vi "PI_AreaScan_Prepare_1.vi"(0 "System":i32 min=0 max=3 step=1, 1 "Laser":string="1", 2 "Axis":string="xy", 3 "da":dbl min=-100.0 max=100.0, 4 "db":dbl min=-100.0 max=100.0, 5 "error in (no error)":errorcluster caption="Fehler (Eingang, kein Fehler)", 6 "a0":dbl=98.0 min=2.0 max=198.0 step=0.01, 8 "b0":dbl min=0.0 max=200.0 step=0.01, 9 "Resolution":dbl=0.01 min=0.01 max=2.0 step=0.01, 10 "c0":dbl min=0.0 max=200.0 step=0.01, 11 "Pixel time":dbl) -> (14 "Tacq":dbl, 15 "lp":i32, 16 "ap":i32, 17 "Trigger":dbl[](array[numeric]), 19 "error out":errorcluster caption="Fehler (Ausgang)")   [LabVIEW 2013]
panel:
  out "ClockDivider":i32
  out "Amplitude":dbl format="%#_3g"
  out "Accelaration":dbl
  out "ttp":i32
  out "Scan lines":dbl
  out "slow axis":i32
  out "fast axis":i32
  out "Colors":i32
  out "Start position":dbl[](array[numeric])
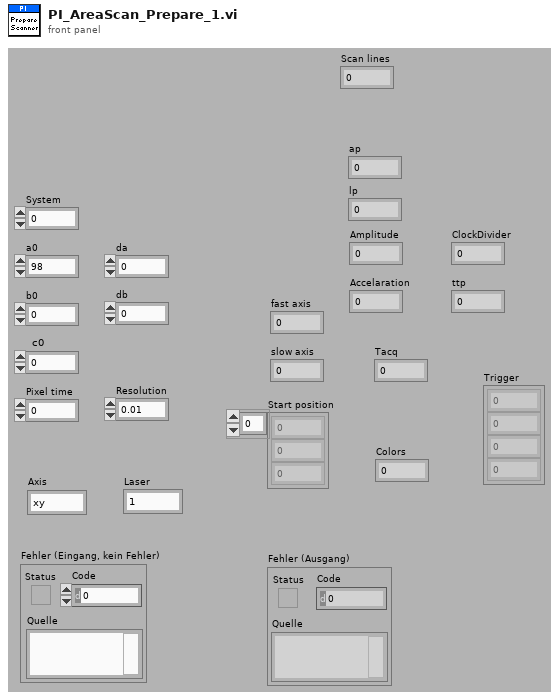
[diagram p1: front panel]
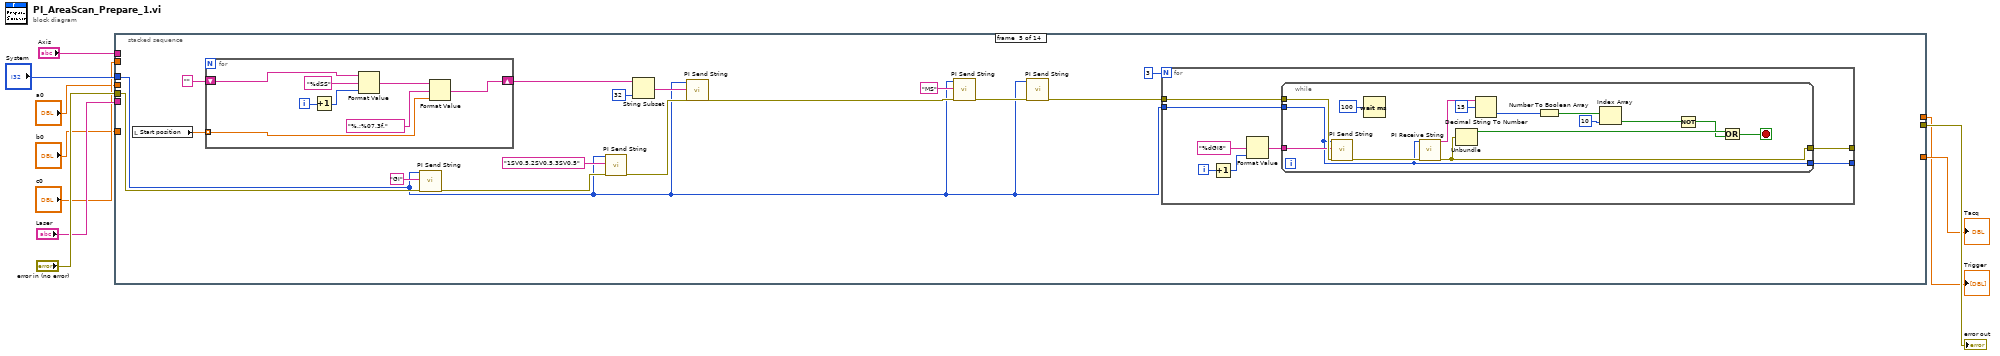
[diagram p0: block diagram]
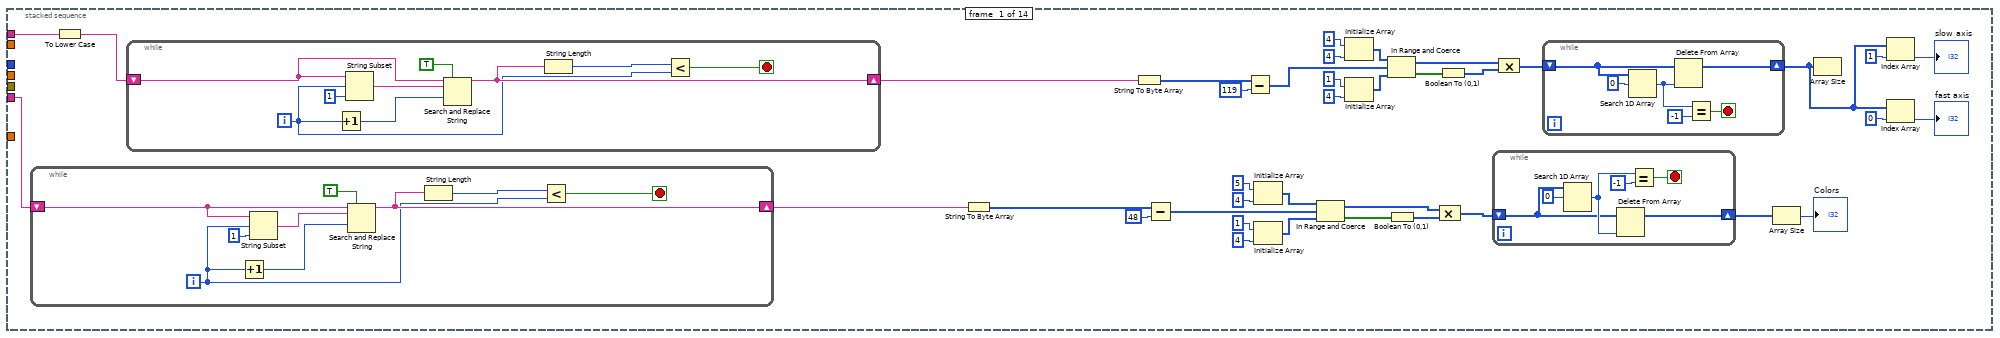
[diagram p2: hidden frame]
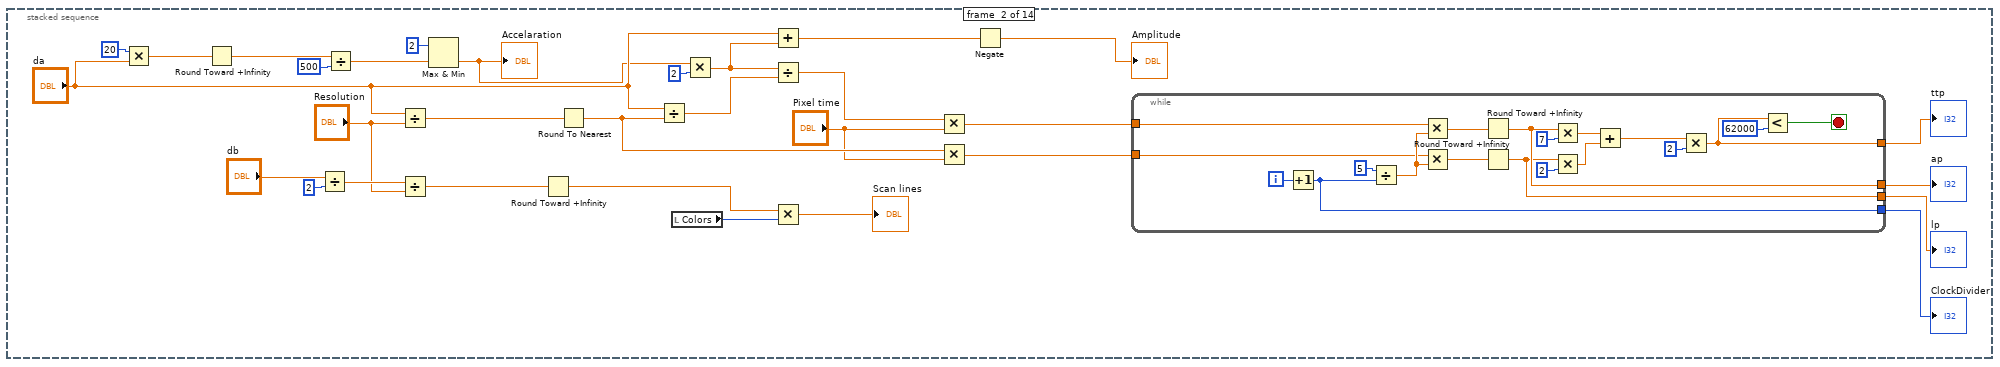
[diagram p3: hidden frame]
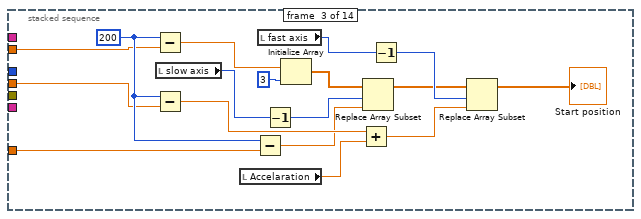
[diagram p4: hidden frame]
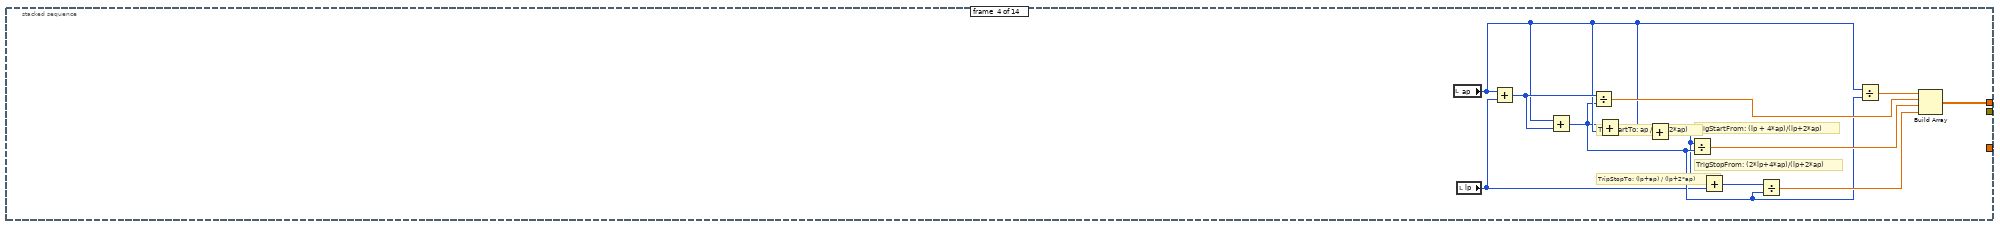
[diagram p5: hidden frame]
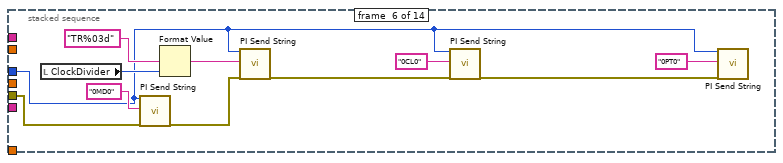
[diagram p6: hidden frame]
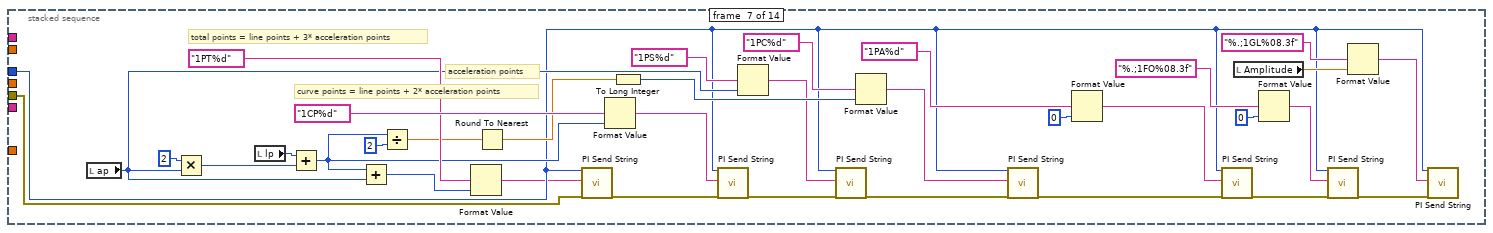
[diagram p7: hidden frame]
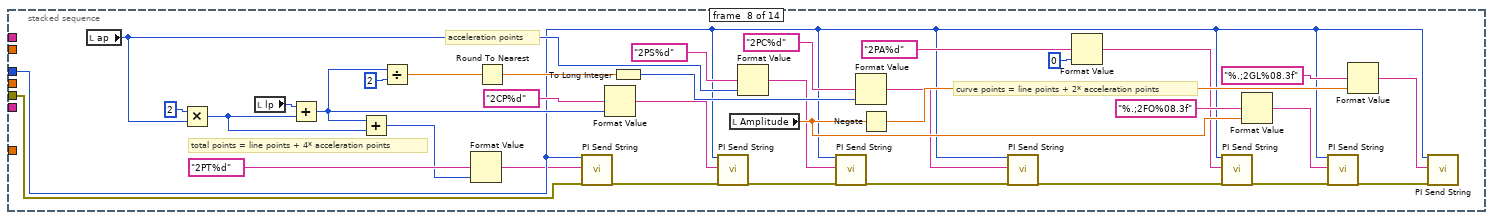
[diagram p8: hidden frame]
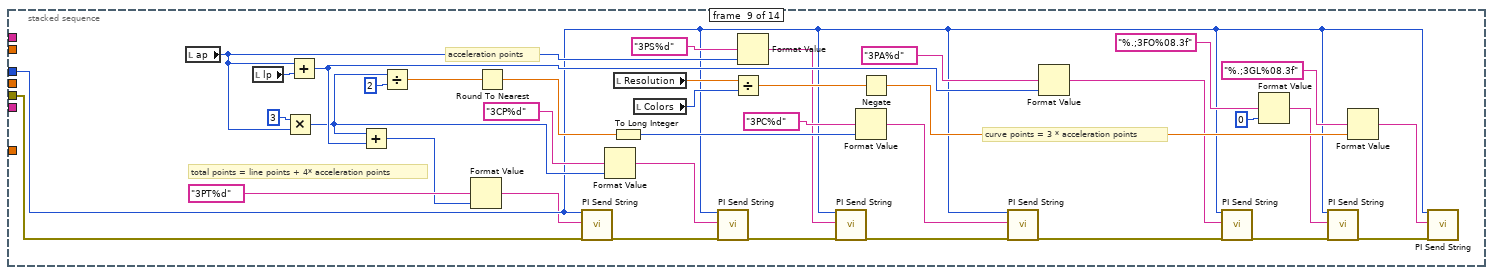
[diagram p9: hidden frame]
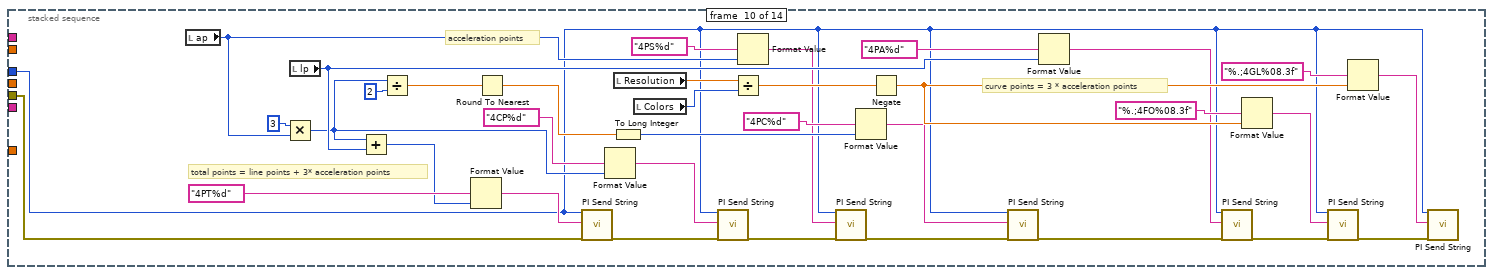
[diagram p10: hidden frame]
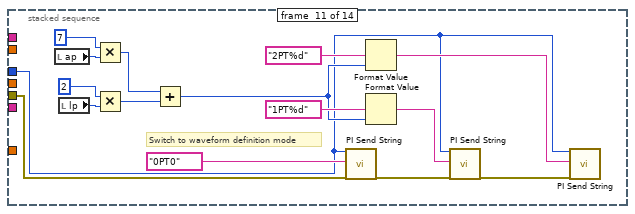
[diagram p11: hidden frame]
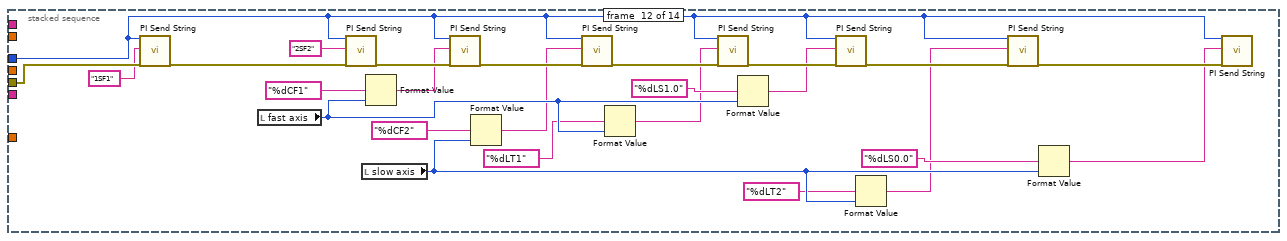
[diagram p12: hidden frame]
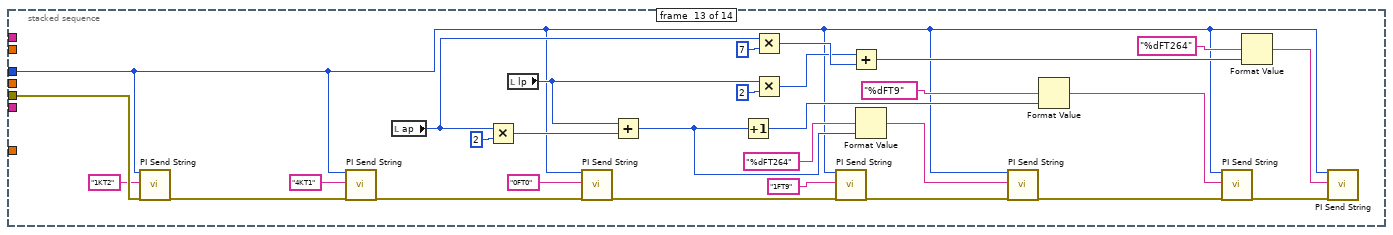
[diagram p13: hidden frame]
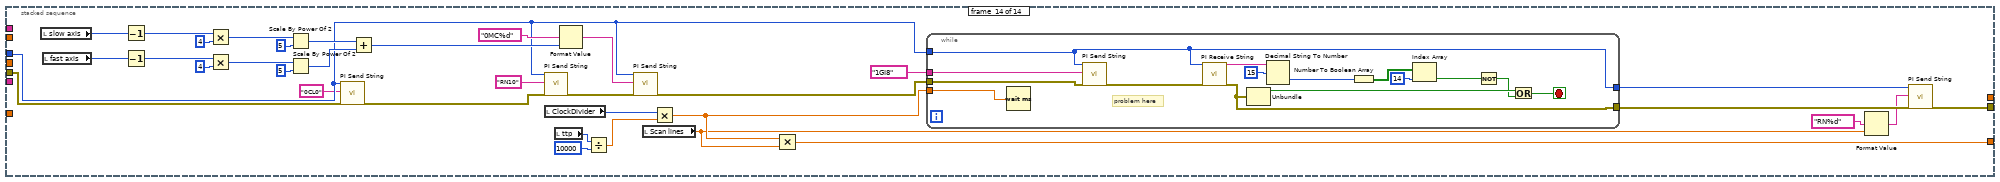
[diagram p14: hidden frame]
diagram:
  n1 = stacked-sequence {
    tunnel: "System" -> [_ _ _ _ w159 w207 w223 w258 w293 w323 w358 w374 w399 w435]
    tunnel: "error in (no error)" -> [_ _ _ _ w167 w212 w224 w265 w300 w331 w362 w390 w407 w439]
    tunnel: [_ _ _ _ _ _ _ _ _ _ _ _ _ w428] -> w8
    tunnel: "Laser" -> [w12 _ _ _ _ _ _ _ _ _ _ _ _ _]
    tunnel: "Axis" -> [w11 _ _ _ _ _ _ _ _ _ _ _ _ _]
    tunnel: "c0" -> [_ _ w131 _ _ _ _ _ _ _ _ _ _ _]
    tunnel: "b0" -> [_ _ w130 _ _ _ _ _ _ _ _ _ _ _]
    tunnel: "a0" -> [_ _ w129 _ _ _ _ _ _ _ _ _ _ _]
    tunnel: [_ _ _ _ _ _ _ _ _ _ _ _ _ w440] -> w2
    tunnel: [_ _ _ w146 _ _ _ _ _ _ _ _ _ _] -> w1
    frame #0 {
      n2 = while {
        shift-right: [w74] -> w39
        shift-left: w12 -> [w78]
        i -> [w70]
        stop <- w73 stop-if-true
        n3 = Increment(x=w70) -> (x+1=w71:i32)
        n4 = String Subset(string=w78, offset (0)=w70, length (rest)=1) -> (substring=w76:string)
        n5 = Search and Replace String(replace all?=TRUE, input string=w78, search string=w76, offset=w71) -> (result string=w74:string)  [unwired: 4 in, 3 out]
        n6 = String Length(string=w74) -> (length=w72:i32)
        n7 = Less?(x=w72, y=w70) -> (x < y?=w73:bool)
      }
      n8 = To Lower Case(string=w11) -> (all lower case string=w19:string)
      n9 = while {
        shift-right: [w59] -> w24
        shift-left: w19 -> [w63]
        i -> [w55]
        stop <- w58 stop-if-true
        n10 = Increment(x=w55) -> (x+1=w56:i32)
        n11 = String Subset(string=w63, offset (0)=w55, length (rest)=1) -> (substring=w61:string)
        n12 = Search and Replace String(replace all?=TRUE, input string=w63, search string=w61, offset=w56) -> (result string=w59:string)  [unwired: 4 in, 3 out]
        n13 = String Length(string=w59) -> (length=w57:i32)
        n14 = Less?(x=w57, y=w55) -> (x < y?=w58:bool)
      }
      n15 = String To Byte Array(string=w39) -> (unsigned byte array=w41:u8[])
      n16 = String To Byte Array(string=w24) -> (unsigned byte array=w26:u8[])
      n17 = Subtract(x=w41, y=48) -> (x-y=w38:i32[])
      n18 = Subtract(x=w26, y=119) -> (x-y=w23:i32[])
      n19 = Initialize Array(5, 4) -> (w46:i32[])
      n20 = Initialize Array(1, 4) -> (w43:i32[])
      n21 = In Range and Coerce(upper limit=w46, x=w38, lower limit=w43) -> (coerced(x)=w35:i32[], In Range?=w42:bool[])
      n22 = Initialize Array(4, 4) -> (w31:i32[])
      n23 = Initialize Array(1, 4) -> (w28:i32[])
      n24 = In Range and Coerce(upper limit=w31, x=w23, lower limit=w28) -> (coerced(x)=w20:i32[], In Range?=w27:bool[])
      n25 = Boolean To (0,1)(Boolean=w42) -> (0, 1=w36:i16[])
      n26 = Boolean To (0,1)(Boolean=w27) -> (0, 1=w21:i16[])
      n27 = Compound Arithmetic op=MULTIPLY(w35, w36) -> (w37:i32[])
      n28 = while {
        shift-right: [w66] -> w34
        shift-left: w37 -> [w64]
        stop <- w67 stop-if-true
        n29 = Search 1D Array(1D array=w64, element=0) -> (index of element=w68:i32)  [unwired: 1 in]
        n30 = Delete From Array(array=w64, index=w68) -> (array with subset deleted=w66:i32[])  [unwired: 1 in, 1 out]
        n31 = Equal?(x=w68, y=-1) -> (x = y?=w67:bool)
      }
      n32 = Compound Arithmetic op=MULTIPLY(w20, w21) -> (w22:i32[])
      n33 = while {
        shift-right: [w51] -> w16
        shift-left: w22 -> [w49]
        stop <- w52 stop-if-true
        n34 = Search 1D Array(1D array=w49, element=0) -> (index of element=w53:i32)  [unwired: 1 in]
        n35 = Delete From Array(array=w49, index=w53) -> (array with subset deleted=w51:i32[])  [unwired: 1 in, 1 out]
        n36 = Equal?(x=w53, y=-1) -> (x = y?=w52:bool)
      }
      n37 = Array Size(array=w34) -> (size(s)=→"Colors":i32)
      n38 = Array Size(array=w16) -> ()  [unwired: 1 out]
      n39 = Index Array(array=w16, index=1) -> (element=→"slow axis":i32)
      n40 = Index Array(array=w16, index=0) -> (element=→"fast axis":i32)
    }
    frame #1 {
      n41 = Multiply(x=20, y="da") -> (x*y=w108:dbl)
      n42 = Round Toward +Infinity(x=w108) -> (ceil(x): smallest int >= x=w107:dbl)
      n43 = Divide(x="db", y=2) -> (x/y=w101:dbl)
      n44 = Divide(x=w107, y=500) -> (x/y=w105:dbl)
      n45 = Divide(x="da", y="Resolution") -> (x/y=w103:dbl)
      n46 = Divide(x=w101, y="Resolution") -> (x/y=w95:dbl)
      n47 = Max & Min(x=2, y=w105) -> (min(x,y)=w86:dbl)  [unwired: 1 out]
      "Accelaration" <- w86
      n48 = Round Toward +Infinity(x=w95) -> (ceil(x): smallest int >= x=w96:dbl)
      n49 = Round To Nearest(number=w103) -> (nearest integer value=w90:dbl)
      n50 = Divide(x="da", y=w90) -> (x/y=w89:dbl)
      n51 = local read "Colors"() -> (w98:i32)
      n52 = Multiply(x=w86, y=2) -> (x*y=w88:dbl)
      n53 = Add(x="da", y=w88) -> (x+y=w80:dbl)
      n54 = Divide(x=w88, y=w89) -> (x/y=w91:dbl)
      n55 = Multiply(x=w96, y=w98) -> (x*y=→"Scan lines":dbl)
      n56 = Multiply(x=w91, y="Pixel time") -> (x*y=w92:dbl)
      n57 = Multiply(x=w90, y="Pixel time") -> (x*y=w94:dbl)
      n58 = Negate(x=w80) -> (-x=→"Amplitude":dbl)
      n59 = while {
        tunnel: w94 -> [w125]
        tunnel: w92 -> [w124]
        tunnel: [w113] -> w84
        tunnel: [w112] -> w81
        tunnel: [w111] -> w83
        tunnel: [w110] -> w82
        i -> [w128]
        stop <- w114 stop-if-true
        n60 = Increment(x=w128) -> (x+1=w112:i32)
        n61 = Divide(x=5, y=w112) -> (x/y=w126:dbl)
        n62 = Multiply(x=w124, y=w126) -> (x*y=w123:dbl)
        n63 = Multiply(x=w125, y=w126) -> (x*y=w122:dbl)
        n64 = Round Toward +Infinity(x=w123) -> (ceil(x): smallest int >= x=w111:dbl)
        n65 = Round Toward +Infinity(x=w122) -> (ceil(x): smallest int >= x=w110:dbl)
        n66 = Multiply(x=w111, y=7) -> (x*y=w119:dbl)
        n67 = Multiply(x=w110, y=2) -> (x*y=w118:dbl)
        n68 = Add(x=w119, y=w118) -> (x+y=w117:dbl)
        n69 = Multiply(x=w117, y=2) -> (x*y=w113:dbl)
        n70 = Less?(x=w113, y=62000) -> (x < y?=w114:bool)
      }
      "ttp" <- w84
      "ap" <- w83
      "lp" <- w82
      "ClockDivider" <- w81
    }
    frame #2 {
      w132 = 200
      n71 = Subtract(x=w132, y=w131) -> (x-y=w134:dbl)
      n72 = Subtract(x=w132, y=w129) -> (x-y=w140:dbl)
      n73 = local read "slow axis"() -> (w145:i32)
      n74 = local read "Accelaration"() -> (w142:dbl)
      n75 = Subtract(x=w132, y=w130) -> (x-y=w136:dbl)
      n76 = local read "fast axis"() -> (w144:i32)
      n77 = Decrement(x=w145) -> (x-1=w138:i32)
      n78 = Initialize Array(w134, 3) -> (w135:dbl[])
      n79 = Add(x=w140, y=w142) -> (x+y=w141:dbl)
      n80 = Replace Array Subset(array=w135, new element=w136, index=w138) -> (w137:dbl[])
      n81 = Decrement(x=w144) -> (x-1=w139:i32)
      n82 = Replace Array Subset(array=w137, new element=w141, index=w139) -> (→"Start position":dbl[])
    }
    frame #3 {
      # "TrigStopFrom: (2*lp+4*ap)/(lp+2*ap)"
      # "TrigStartFrom: (lp + 4*ap)/(lp+2*ap)"
      # "TripStopTo: (lp+ap) / (lp+2*ap)"
      # "TrigStartTo: ap / (lp+2*ap)"
      n83 = local read "ap"() -> (w152:i32)
      n84 = local read "lp"() -> (w148:i32)
      n85 = Add(x=w152, y=w148) -> (x+y=w153:i32)
      n86 = Add(x=w152, y=w153) -> (x+y=w151:i32)
      n87 = Divide(x=w153, y=w151) -> (x/y=w155:dbl)
      n88 = Add(x=w151, y=w152) -> (x+y=w150:i32)
      n89 = Add(x=w150, y=w152) -> (x+y=w147:i32)
      n90 = Divide(x=w147, y=w151) -> (x/y=w156:dbl)
      n91 = Add(x=w147, y=w148) -> (x+y=w149:i32)
      n92 = Divide(x=w149, y=w151) -> (x/y=w157:dbl)
      n93 = Divide(x=w152, y=w151) -> (x/y=w154:dbl)
      n94 = Build Array(w154, w155, w156, w157) -> (w146:dbl[])
    }
    frame #4 {
      n95 = local read "Start position"() -> (w171:dbl[])
      n96 = for {
        shift-right: [w202] -> w172
        shift-left: "" -> [w204]
        tunnel: w171 -> [w197] mode=indexing
        i -> [w199]
        n97 = Increment(x=w199) -> (x+1=w198:i32)
        n98 = Format Value(string ("")=w204, format string="%dSS", value (0)=w198) -> (output string=w203:string)
        n99 = Format Value(string ("")=w203, format string="%.;%07.3f,", value (0)=w197) -> (output string=w202:string)
      }
      n100 = call "PI Send String.vi"("System no."=w159, "String to send"="GI", "error in"=w167) -> ("error out"=w166:errorcluster)  [unwired: 16 in]
      n101 = call "PI Send String.vi"("System no."=w159, "String to send"="1SV0.5,2SV0.5,3SV0.5", "error in"=w166) -> ("error out"=w163:errorcluster)  [unwired: 16 in]
      n102 = String Subset(string=w172, length (rest)=32) -> (substring=w164:string)  [unwired: 1 in]
      n103 = call "PI Send String.vi"("System no."=w159, "String to send"=w164, "error in"=w163) -> ("error out"=w161:errorcluster)  [unwired: 16 in]
      n104 = call "PI Send String.vi"("System no."=w159, "String to send"="MS", "error in"=w161) -> ("error out"=w160:errorcluster)  [unwired: 16 in]
      n105 = call "PI Send String.vi"("System no."=w159, "error in"=w160) -> ("error out"=w158:errorcluster)  [unwired: 17 in]
      n106 = for {
        N: 3 -> [_]
        tunnel: w158 -> [w177]
        tunnel: w159 -> [w176]
        tunnel: [w175] -> _
        tunnel: [w174] -> _
        i -> [w181]
        n107 = Increment(x=w181) -> (x+1=w180:i32)
        n108 = Format Value(format string="%dGI8", value (0)=w180) -> (output string=w178:string)  [unwired: 1 in]
        n109 = while {
          tunnel: w178 -> [w186]
          tunnel: w177 -> [w187]
          tunnel: w176 -> [w184]
          tunnel: [w182] -> w175
          tunnel: [w184] -> w174
          stop <- w190 stop-if-true
          n110 = call "PI Send String.vi"("System no."=w184, "String to send"=w186, "error in"=w187) -> ("error out"=w185:errorcluster)  [unwired: 16 in]
          n111 = Wait (ms)(milliseconds to wait=100) -> ()  [unwired: 1 out]
          n112 = call "PI Receive String.vi"("System no."=w184, "error in"=w185) -> ("String read"=w183:string, "error out"=w182:errorcluster)  [unwired: 15 in, 1 out]
          n113 = Unbundle(w182) -> ("status"=w194:bool)  [unwired: 2 out]
          n114 = Decimal String To Number(string=w183, offset=15) -> (number=w195:i32)  [unwired: 1 in, 1 out]
          n115 = Number To Boolean Array(number=w195) -> (Boolean array=w192:bool[])
          n116 = Index Array(array=w192, index=10) -> (element=w191:bool)
          n117 = Not(x=w191) -> (.not. x?=w188:bool)
          n118 = Or(x=w194, y=w188) -> (x .or. y?=w190:bool)
        }
      }
    }
    frame #5 {
      n119 = local read "ClockDivider"() -> (w215:i32)
      n120 = call "PI Send String.vi"("System no."=w207, "String to send"="0MD0", "error in"=w212) -> ("error out"=w211:errorcluster)  [unwired: 16 in]
      n121 = Format Value(format string="TR%03d", value (0)=w215) -> (output string=w206:string)  [unwired: 1 in]
      n122 = call "PI Send String.vi"("System no."=w207, "String to send"=w206, "error in"=w211) -> ("error out"=w210:errorcluster)  [unwired: 16 in]
      n123 = call "PI Send String.vi"("System no."=w207, "String to send"="0CL0", "error in"=w210) -> ("error out"=w209:errorcluster)  [unwired: 16 in]
      n124 = call "PI Send String.vi"("System no."=w207, "String to send"="0PT0", "error in"=w209) -> ()  [unwired: 16 in, 1 out]
    }
    frame #6 {
      # "acceleration points"
      # "total points = line points + 3* acceleration points"
      # "curve points = line points + 2* acceleration points"
      n125 = local read "ap"() -> (w239:i32)
      n126 = Multiply(x=2, y=w239) -> (x*y=w242:i32)
      n127 = local read "lp"() -> (w241:i32)
      n128 = Add(x=w241, y=w242) -> (x+y=w236:i32)
      n129 = Add(x=w236, y=w239) -> (x+y=w240:i32)
      n130 = Divide(x=w236, y=2) -> (x/y=w235:dbl)
      n131 = Format Value(format string="1PT%d", value (0)=w240) -> (output string=w222:string)  [unwired: 1 in]
      n132 = Round To Nearest(number=w235) -> (nearest integer value=w232:dbl)
      n133 = call "PI Send String.vi"("System no."=w223, "String to send"=w222, "error in"=w224) -> ("error out"=w230:errorcluster)  [unwired: 16 in]
      n134 = Format Value(format string="1CP%d", value (0)=w236) -> (output string=w221:string)  [unwired: 1 in]
      n135 = To Long Integer(number=w232) -> (32bit integer=w233:i32)
      n136 = call "PI Send String.vi"("System no."=w223, "String to send"=w221, "error in"=w230) -> ("error out"=w229:errorcluster)  [unwired: 16 in]
      n137 = Format Value(format string="1PS%d", value (0)=w239) -> (output string=w220:string)  [unwired: 1 in]
      n138 = call "PI Send String.vi"("System no."=w223, "String to send"=w220, "error in"=w229) -> ("error out"=w228:errorcluster)  [unwired: 16 in]
      n139 = Format Value(format string="1PC%d", value (0)=w233) -> (output string=w219:string)  [unwired: 1 in]
      n140 = call "PI Send String.vi"("System no."=w223, "String to send"=w219, "error in"=w228) -> ("error out"=w227:errorcluster)  [unwired: 16 in]
      n141 = Format Value(format string="1PA%d", value (0)=0) -> (output string=w218:string)  [unwired: 1 in]
      n142 = call "PI Send String.vi"("System no."=w223, "String to send"=w218, "error in"=w227) -> ("error out"=w226:errorcluster)  [unwired: 16 in]
      n143 = local read "Amplitude"() -> (w231:dbl)
      n144 = Format Value(format string="%.;1FO%08.3f", value (0)=0) -> (output string=w217:string)  [unwired: 1 in]
      n145 = call "PI Send String.vi"("System no."=w223, "String to send"=w217, "error in"=w226) -> ("error out"=w225:errorcluster)  [unwired: 16 in]
      n146 = Format Value(format string="%.;1GL%08.3f", value (0)=w231) -> (output string=w216:string)  [unwired: 1 in]
      n147 = call "PI Send String.vi"("System no."=w223, "String to send"=w216, "error in"=w225) -> ()  [unwired: 16 in, 1 out]
    }
    frame #7 {
      # "acceleration points"
      # "total points = line points + 4* acceleration points"
      # "curve points = line points + 2* acceleration points"
      n148 = local read "ap"() -> (w276:i32)
      n149 = Multiply(x=2, y=w276) -> (x*y=w275:i32)
      n150 = local read "lp"() -> (w278:i32)
      n151 = Add(x=w278, y=w275) -> (x+y=w269:i32)
      n152 = Add(x=w269, y=w275) -> (x+y=w277:i32)
      n153 = Divide(x=w269, y=2) -> (x/y=w273:dbl)
      n154 = Format Value(format string="2PT%d", value (0)=w277) -> (output string=w257:string)  [unwired: 1 in]
      n155 = Round To Nearest(number=w273) -> (nearest integer value=w270:dbl)
      n156 = call "PI Send String.vi"("System no."=w258, "String to send"=w257, "error in"=w265) -> ("error out"=w264:errorcluster)  [unwired: 16 in]
      n157 = Format Value(format string="2CP%d", value (0)=w269) -> (output string=w256:string)  [unwired: 1 in]
      n158 = To Long Integer(number=w270) -> (32bit integer=w271:i32)
      n159 = call "PI Send String.vi"("System no."=w258, "String to send"=w256, "error in"=w264) -> ("error out"=w263:errorcluster)  [unwired: 16 in]
      n160 = local read "Amplitude"() -> (w267:dbl)
      n161 = Format Value(format string="2PS%d", value (0)=w276) -> (output string=w255:string)  [unwired: 1 in]
      n162 = call "PI Send String.vi"("System no."=w258, "String to send"=w255, "error in"=w263) -> ("error out"=w262:errorcluster)  [unwired: 16 in]
      n163 = Format Value(format string="2PC%d", value (0)=w271) -> (output string=w254:string)  [unwired: 1 in]
      n164 = Negate(x=w267) -> (-x=w266:dbl)
      n165 = call "PI Send String.vi"("System no."=w258, "String to send"=w254, "error in"=w262) -> ("error out"=w261:errorcluster)  [unwired: 16 in]
      n166 = Format Value(format string="2PA%d", value (0)=0) -> (output string=w253:string)  [unwired: 1 in]
      n167 = call "PI Send String.vi"("System no."=w258, "String to send"=w253, "error in"=w261) -> ("error out"=w260:errorcluster)  [unwired: 16 in]
      n168 = Format Value(format string="%.;2FO%08.3f", value (0)=w267) -> (output string=w252:string)  [unwired: 1 in]
      n169 = call "PI Send String.vi"("System no."=w258, "String to send"=w252, "error in"=w260) -> ("error out"=w259:errorcluster)  [unwired: 16 in]
      n170 = Format Value(format string="%.;2GL%08.3f", value (0)=w266) -> (output string=w251:string)  [unwired: 1 in]
      n171 = call "PI Send String.vi"("System no."=w258, "String to send"=w251, "error in"=w259) -> ()  [unwired: 16 in, 1 out]
    }
    frame #8 {
      # "acceleration points"
      # "total points = line points + 4* acceleration points"
      # "curve points = 3 * acceleration points"
      n172 = local read "ap"() -> (w307:i32)
      n173 = local read "lp"() -> (w310:i32)
      n174 = Multiply(x=3, y=w307) -> (x*y=w302:i32)
      n175 = Add(x=w307, y=w310) -> (x+y=w308:i32)
      n176 = Add(x=w302, y=w308) -> (x+y=w316:i32)
      n177 = Divide(x=w302, y=2) -> (x/y=w306:dbl)
      n178 = Format Value(format string="3PT%d", value (0)=w316) -> (output string=w292:string)  [unwired: 1 in]
      n179 = Round To Nearest(number=w306) -> (nearest integer value=w303:dbl)
      n180 = call "PI Send String.vi"("System no."=w293, "String to send"=w292, "error in"=w300) -> ("error out"=w299:errorcluster)  [unwired: 16 in]
      n181 = Format Value(format string="3CP%d", value (0)=w302) -> (output string=w291:string)  [unwired: 1 in]
      n182 = To Long Integer(number=w303) -> (32bit integer=w304:i32)
      n183 = local read "Resolution"() -> (w315:dbl)
      n184 = local read "Colors"() -> (w312:i32)
      n185 = call "PI Send String.vi"("System no."=w293, "String to send"=w291, "error in"=w299) -> ("error out"=w298:errorcluster)  [unwired: 16 in]
      n186 = Divide(x=w315, y=w312) -> (x/y=w313:dbl)
      n187 = Format Value(format string="3PS%d", value (0)=w307) -> (output string=w290:string)  [unwired: 1 in]
      n188 = call "PI Send String.vi"("System no."=w293, "String to send"=w290, "error in"=w298) -> ("error out"=w297:errorcluster)  [unwired: 16 in]
      n189 = Format Value(format string="3PC%d", value (0)=w304) -> (output string=w289:string)  [unwired: 1 in]
      n190 = Negate(x=w313) -> (-x=w311:dbl)
      n191 = call "PI Send String.vi"("System no."=w293, "String to send"=w289, "error in"=w297) -> ("error out"=w296:errorcluster)  [unwired: 16 in]
      n192 = Format Value(format string="3PA%d", value (0)=w308) -> (output string=w288:string)  [unwired: 1 in]
      n193 = call "PI Send String.vi"("System no."=w293, "String to send"=w288, "error in"=w296) -> ("error out"=w295:errorcluster)  [unwired: 16 in]
      n194 = Format Value(format string="%.;3FO%08.3f", value (0)=0) -> (output string=w287:string)  [unwired: 1 in]
      n195 = call "PI Send String.vi"("System no."=w293, "String to send"=w287, "error in"=w295) -> ("error out"=w294:errorcluster)  [unwired: 16 in]
      n196 = Format Value(format string="%.;3GL%08.3f", value (0)=w311) -> (output string=w286:string)  [unwired: 1 in]
      n197 = call "PI Send String.vi"("System no."=w293, "String to send"=w286, "error in"=w294) -> ()  [unwired: 16 in, 1 out]
    }
    frame #9 {
      # "acceleration points"
      # "total points = line points + 3* acceleration points"
      # "curve points = 3 * acceleration points"
      n198 = local read "ap"() -> (w347:i32)
      n199 = Multiply(x=3, y=w347) -> (x*y=w339:i32)
      n200 = local read "lp"() -> (w345:i32)
      n201 = Add(x=w339, y=w345) -> (x+y=w351:i32)
      n202 = Divide(x=w339, y=2) -> (x/y=w343:dbl)
      n203 = Format Value(format string="4PT%d", value (0)=w351) -> (output string=w330:string)  [unwired: 1 in]
      n204 = Round To Nearest(number=w343) -> (nearest integer value=w340:dbl)
      n205 = call "PI Send String.vi"("System no."=w323, "String to send"=w330, "error in"=w331) -> ("error out"=w337:errorcluster)  [unwired: 16 in]
      n206 = Format Value(format string="4CP%d", value (0)=w339) -> (output string=w329:string)  [unwired: 1 in]
      n207 = To Long Integer(number=w340) -> (32bit integer=w341:i32)
      n208 = local read "Resolution"() -> (w350:dbl)
      n209 = local read "Colors"() -> (w349:i32)
      n210 = call "PI Send String.vi"("System no."=w323, "String to send"=w329, "error in"=w337) -> ("error out"=w336:errorcluster)  [unwired: 16 in]
      n211 = Divide(x=w350, y=w349) -> (x/y=w346:dbl)
      n212 = Format Value(format string="4PS%d", value (0)=w347) -> (output string=w328:string)  [unwired: 1 in]
      n213 = call "PI Send String.vi"("System no."=w323, "String to send"=w328, "error in"=w336) -> ("error out"=w335:errorcluster)  [unwired: 16 in]
      n214 = Format Value(format string="4PC%d", value (0)=w341) -> (output string=w327:string)  [unwired: 1 in]
      n215 = Negate(x=w346) -> (-x=w344:dbl)
      n216 = call "PI Send String.vi"("System no."=w323, "String to send"=w327, "error in"=w335) -> ("error out"=w334:errorcluster)  [unwired: 16 in]
      n217 = Format Value(format string="4PA%d", value (0)=w345) -> (output string=w326:string)  [unwired: 1 in]
      n218 = call "PI Send String.vi"("System no."=w323, "String to send"=w326, "error in"=w334) -> ("error out"=w333:errorcluster)  [unwired: 16 in]
      n219 = Format Value(format string="%.;4FO%08.3f", value (0)=w344) -> (output string=w325:string)  [unwired: 1 in]
      n220 = call "PI Send String.vi"("System no."=w323, "String to send"=w325, "error in"=w333) -> ("error out"=w332:errorcluster)  [unwired: 16 in]
      n221 = Format Value(format string="%.;4GL%08.3f", value (0)=w344) -> (output string=w324:string)  [unwired: 1 in]
      n222 = call "PI Send String.vi"("System no."=w323, "String to send"=w324, "error in"=w332) -> ()  [unwired: 16 in, 1 out]
    }
    frame #10 {
      # "Switch to waveform definition mode"
      n223 = local read "ap"() -> (w370:i32)
      n224 = local read "lp"() -> (w371:i32)
      n225 = Multiply(x=7, y=w370) -> (x*y=w367:i32)
      n226 = Multiply(x=2, y=w371) -> (x*y=w366:i32)
      n227 = Add(x=w367, y=w366) -> (x+y=w365:i32)
      n228 = call "PI Send String.vi"("System no."=w358, "String to send"="0PT0", "error in"=w362) -> ("error out"=w364:errorcluster)  [unwired: 16 in]
      n229 = Format Value(format string="2PT%d", value (0)=w365) -> (output string=w359:string)  [unwired: 1 in]
      n230 = Format Value(format string="1PT%d", value (0)=w365) -> (output string=w360:string)  [unwired: 1 in]
      n231 = call "PI Send String.vi"("System no."=w358, "String to send"=w360, "error in"=w364) -> ("error out"=w363:errorcluster)  [unwired: 16 in]
      n232 = call "PI Send String.vi"("System no."=w358, "String to send"=w359, "error in"=w363) -> ()  [unwired: 16 in, 1 out]
    }
    frame #11 {
      n233 = call "PI Send String.vi"("System no."=w374, "String to send"="1SF1", "error in"=w390) -> ("error out"=w389:errorcluster)  [unwired: 16 in]
      n234 = local read "fast axis"() -> (w398:i32)
      n235 = call "PI Send String.vi"("System no."=w374, "String to send"="2SF2", "error in"=w389) -> ("error out"=w388:errorcluster)  [unwired: 16 in]
      n236 = local read "slow axis"() -> (w397:i32)
      n237 = Format Value(format string="%dCF1", value (0)=w398) -> (output string=w380:string)  [unwired: 1 in]
      n238 = call "PI Send String.vi"("System no."=w374, "String to send"=w380, "error in"=w388) -> ("error out"=w387:errorcluster)  [unwired: 16 in]
      n239 = Format Value(format string="%dCF2", value (0)=w397) -> (output string=w379:string)  [unwired: 1 in]
      n240 = call "PI Send String.vi"("System no."=w374, "String to send"=w379, "error in"=w387) -> ("error out"=w386:errorcluster)  [unwired: 16 in]
      n241 = Format Value(format string="%dLT1", value (0)=w398) -> (output string=w378:string)  [unwired: 1 in]
      n242 = call "PI Send String.vi"("System no."=w374, "String to send"=w378, "error in"=w386) -> ("error out"=w385:errorcluster)  [unwired: 16 in]
      n243 = Format Value(format string="%dLS1.0", value (0)=w398) -> (output string=w377:string)  [unwired: 1 in]
      n244 = call "PI Send String.vi"("System no."=w374, "String to send"=w377, "error in"=w385) -> ("error out"=w384:errorcluster)  [unwired: 16 in]
      n245 = Format Value(format string="%dLT2", value (0)=w397) -> (output string=w376:string)  [unwired: 1 in]
      n246 = call "PI Send String.vi"("System no."=w374, "String to send"=w376, "error in"=w384) -> ("error out"=w383:errorcluster)  [unwired: 16 in]
      n247 = Format Value(format string="%dLS0.0", value (0)=w397) -> (output string=w375:string)  [unwired: 1 in]
      n248 = call "PI Send String.vi"("System no."=w374, "String to send"=w375, "error in"=w383) -> ()  [unwired: 16 in, 1 out]
    }
    frame #12 {
      n249 = call "PI Send String.vi"("System no."=w399, "String to send"="1KT2", "error in"=w407) -> ("error out"=w413:errorcluster)  [unwired: 16 in]
      n250 = call "PI Send String.vi"("System no."=w399, "String to send"="4KT1", "error in"=w413) -> ("error out"=w412:errorcluster)  [unwired: 16 in]
      n251 = local read "ap"() -> (w422:i32)
      n252 = Multiply(x=w422, y=2) -> (x*y=w425:i32)
      n253 = local read "lp"() -> (w420:i32)
      n254 = call "PI Send String.vi"("System no."=w399, "String to send"="0FT0", "error in"=w412) -> ("error out"=w411:errorcluster)  [unwired: 16 in]
      n255 = Add(x=w420, y=w425) -> (x+y=w414:i32)
      n256 = Increment(x=w414) -> (x+1=w415:i32)
      n257 = Multiply(x=w422, y=7) -> (x*y=w419:i32)
      n258 = Multiply(x=w420, y=2) -> (x*y=w418:i32)
      n259 = call "PI Send String.vi"("System no."=w399, "String to send"="1FT9", "error in"=w411) -> ("error out"=w410:errorcluster)  [unwired: 16 in]
      n260 = Add(x=w418, y=w419) -> (x+y=w417:i32)
      n261 = Format Value(format string="%dFT264", value (0)=w414) -> (output string=w402:string)  [unwired: 1 in]
      n262 = call "PI Send String.vi"("System no."=w399, "String to send"=w402, "error in"=w410) -> ("error out"=w409:errorcluster)  [unwired: 16 in]
      n263 = Format Value(format string="%dFT9", value (0)=w415) -> (output string=w401:string)  [unwired: 1 in]
      n264 = call "PI Send String.vi"("System no."=w399, "String to send"=w401, "error in"=w409) -> ("error out"=w408:errorcluster)  [unwired: 16 in]
      n265 = Format Value(format string="%dFT264", value (0)=w417) -> (output string=w400:string)  [unwired: 1 in]
      n266 = call "PI Send String.vi"("System no."=w399, "String to send"=w400, "error in"=w408) -> ()  [unwired: 16 in, 1 out]
    }
    frame #13 {
      n267 = local read "slow axis"() -> (w462:i32)
      n268 = local read "fast axis"() -> (w461:i32)
      n269 = Decrement(x=w462) -> (x-1=w445:i32)
      n270 = Decrement(x=w461) -> (x-1=w449:i32)
      n271 = Multiply(x=w445, y=4) -> (x*y=w443:i32)
      n272 = Multiply(x=w449, y=4) -> (x*y=w447:i32)
      n273 = Scale By Power Of 2(n=w443, x=u8 5) -> (x*2^n=w450:u8)
      n274 = Scale By Power Of 2(n=w447, x=u8 5) -> (x*2^n=w451:u8)
      n275 = call "PI Send String.vi"("System no."=w435, "String to send"="0CL0", "error in"=w439) -> ("error out"=w438:errorcluster)  [unwired: 16 in]
      n276 = Add(x=w450, y=w451) -> (x+y=w452:u8)
      n277 = call "PI Send String.vi"("System no."=w435, "String to send"="RN10", "error in"=w438) -> ("error out"=w437:errorcluster)  [unwired: 16 in]
      n278 = local read "ClockDivider"() -> (w460:i32)
      n279 = local read "ttp"() -> (w459:i32)
      n280 = Format Value(format string="0MC%d", value (0)=w452) -> (output string=w432:string)  [unwired: 1 in]
      n281 = Divide(x=w459, y=10000) -> (x/y=w454:dbl)
      n282 = call "PI Send String.vi"("System no."=w435, "String to send"=w432, "error in"=w437) -> ("error out"=w436:errorcluster)  [unwired: 16 in]
      n283 = local read "Scan lines"() -> (w456:dbl)
      n284 = Multiply(x=w460, y=w454) -> (x*y=w457:dbl)
      n285 = Multiply(x=w457, y=w456) -> (x*y=w440:dbl)
      n286 = while {
        tunnel: "1GI8" -> [w464]
        tunnel: w436 -> [w466]
        tunnel: w435 -> [w465]
        tunnel: [w467] -> w431
        tunnel: [w465] -> w430
        tunnel: w457 -> [w475]
        stop <- w472 stop-if-true
        # "problem here"
        n287 = Wait (ms)(milliseconds to wait=w475) -> ()  [unwired: 1 out]
        n288 = call "PI Send String.vi"("System no."=w465, "String to send"=w464, "error in"=w466) -> ("error out"=w463:errorcluster)  [unwired: 16 in]
        n289 = call "PI Receive String.vi"("System no."=w465, "error in"=w463) -> ("String read"=w468:string, "error out"=w467:errorcluster)  [unwired: 15 in, 1 out]
        n290 = Unbundle(w467) -> ("status"=w470:bool)  [unwired: 2 out]
        n291 = Decimal String To Number(string=w468, offset=15) -> (number=w476:i32)  [unwired: 1 in, 1 out]
        n292 = Number To Boolean Array(number=w476) -> (Boolean array=w474:bool[])
        n293 = Index Array(array=w474, index=14) -> (element=w471:bool)
        n294 = Not(x=w471) -> (.not. x?=w469:bool)
        n295 = Or(x=w470, y=w469) -> (x .or. y?=w472:bool)
      }
      n296 = Format Value(format string="RN%d", value (0)=w456) -> (output string=w429:string)  [unwired: 1 in]
      n297 = call "PI Send String.vi"("System no."=w430, "String to send"=w429, "error in"=w431) -> ("error out"=w428:errorcluster)  [unwired: 16 in]
    }
  }
  "error out" <- w8
  "Tacq" <- w2
  "Trigger" <- w1
